vi "AuMT8852B EUT Remote Power Control.vi"(7 "Power control (Minimum)":T1(ring), 8 "error in (no error)":errorcluster, 11 "VISA session":refnum<visa-resource-name>) -> (0 "error out":errorcluster, 2 "error code":i32, 3 "VISA session out":refnum<visa-resource-name>)   [LabVIEW 2017]
doc: "Anritsu MT8852B Bluetooth Tester\n\nAlters the state of the EUT TX power if the EUT supports power control.\n\nINPUTS\nPower control - how the EUT power will be adjusted."
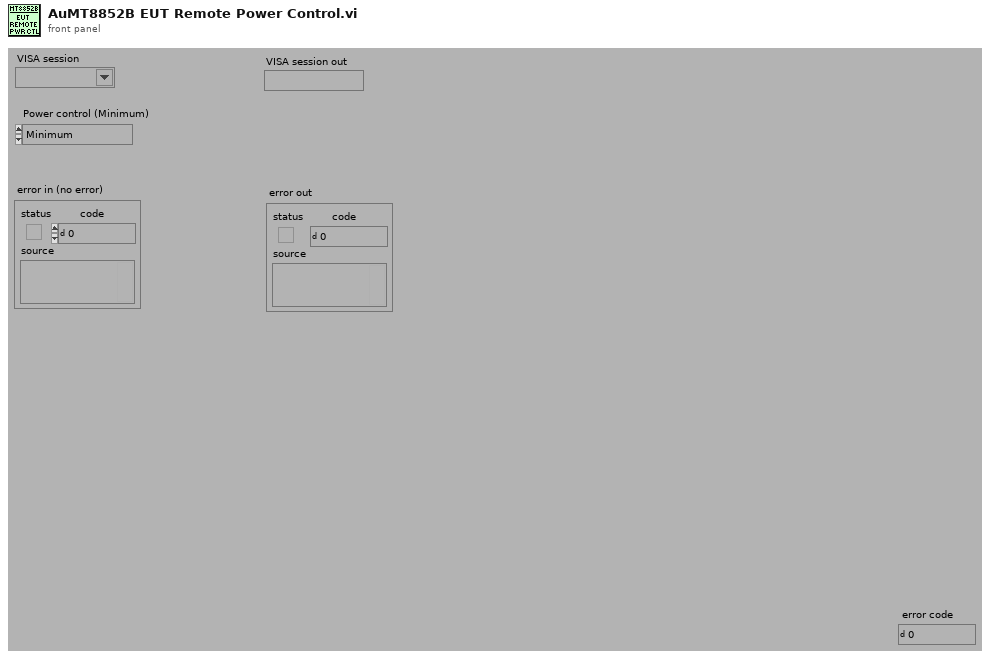
[diagram p1: front panel]
types:
  T1 = enum16{"Minimum", "Decrement", "Increment", "Maximum"}
  T2 = enum16{"Simulate", "Range check", "Cache", "Query instrument status"}
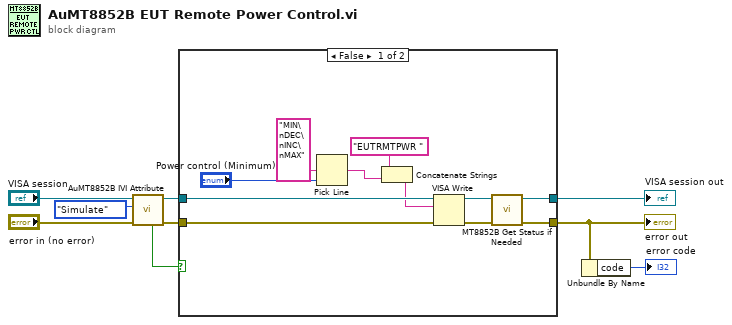
[diagram p0: block diagram]
diagram:
  n1 = call <instrlib>:"AuMT8852B IVI Attribute.vi"("error in (no error)"="error in (no error)", "Flag (Simulate)"=T2."Simulate", "VISA session"="VISA session") -> ("error out"=w5:errorcluster, "VISA session out"=w6:refnum<visa-resource-name>, "Value out"=w4:bool)  [unwired: 6 in]
  n2 = case shown="False" w4 {
    tunnel: [w15 w21] -> w7
    tunnel: [w16 w22] -> w9
    tunnel: w6 -> [w20 w22]
    tunnel: w5 -> [w19 w21]
    frame False {
      n3 = Pick Line(multi-line string="MIN\nDEC\nINC\nMAX", line index="Power control (Minimum)") -> (output string=w10:string)  [unwired: 1 in]
      n4 = Concatenate Strings("EUTRMTPWR " ("Format String"), w10) -> (w13:string)
      n5 = VISA Write(VISA resource name=w20, write buffer=w13, error in (no error)=w19) -> (VISA resource name out=w18:refnum<visa-resource-name>, error out=w17:errorcluster)  [unwired: 1 out]
      n6 = call <instrlib>:"MT8852B Get Status if Needed.vi"("error in (no error)"=w17, "VISA session"=w18) -> ("error out"=w15:errorcluster, "VISA session out"=w16:refnum<visa-resource-name>)  [unwired: 8 in]
    }
    frame True {
    }
  }
  "error out" <- w7
  "VISA session out" <- w9
  n7 = Unbundle By Name(w7) -> ("code"=→"error code":i32)
